vi "NISE.remote.init request string.vi"(8 "error in (no error)":errorcluster, 10 "slsc type":T1, 11 "resource":string) -> (0 "error out":errorcluster, 3 "Request String":string)   [LabVIEW 2016, in "SLSC Interface.lvclass"]
uses:
  SLSC Interface Class/SLSC Interface.lvclass
  SLSC Interface Class/NISE.slsc type.ctl
  <vilib>/NI/JSON Support for LabVIEW/JSON Data Classes/JSON Object/JSON Object.lvclass
  C:/Program Files (x86)/National Instruments/LabVIEW 2016/vi.lib/NI/JSON Support for LabVIEW/JSON Data Classes/JSON Datatype/JSON Null.lvclass
  <vilib>/NI/JSON Support for LabVIEW/JSON Data Classes/JSON Object/New JSON Object (Empty).vi
  <vilib>/NI/JSON Support for LabVIEW/JSON Data Classes/JSON Object/Insert Key Value Pair (Single String).vi
  <vilib>/NI/NI JSONRPC Server Framework/Classes/Server/Format Client Request (Auto-Increment).vi
  <vilib>/NI/NI JSONRPC Server Framework/Classes/Server/JSONRPC Server.lvclass
  <vilib>/NI/JSON Support for LabVIEW/JSON Data Classes/JSON Helper/JSON Helper.lvclass
  C:/Program Files (x86)/National Instruments/LabVIEW 2016/vi.lib/NI/JSON Support for LabVIEW/JSON Data Classes/JSON Structured Type/JSON Structure.lvclass
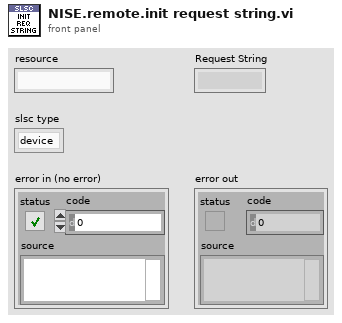
[diagram p1: front panel]
types:
  T1 = typedef "SLSC Interface.lvclass/NISE.slsc type.ctl" = enum16{"device", "nvmem", "channel", "none"}
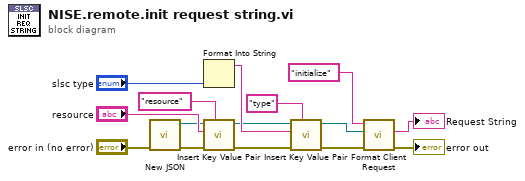
[diagram p0: block diagram]
diagram:
  n1 = call-poly <vilib>:"New JSON.vi"("error in (no error)"="error in (no error)") -> ("error out"=w9:errorcluster, "JSON Object out"=w2:refnum<class "JSON Object.lvclass">)  [unwired: 9 in]
  n2 = Format Into String("slsc type") -> (resulting string=w3:string)  [unwired: 3 in, 1 out]
  n3 = call-poly <vilib>:"Insert Key Value Pair.vi"("key"="resource" ("Name"), "error in (no error)"=w9, "value"="resource", "JSON Object in"=w2) -> ("error out"=w8:errorcluster, "JSON Object out"=w1:refnum<class "JSON Object.lvclass">)  [unwired: 5 in, 1 out]
  n4 = call-poly <vilib>:"Insert Key Value Pair.vi"("key"="type" ("Name"), "error in (no error)"=w8, "value"=w3, "JSON Object in"=w1) -> ("error out"=w12:errorcluster, "JSON Object out"=w10:refnum<class "JSON Object.lvclass">)  [unwired: 5 in, 1 out]
  n5 = call-poly <vilib>:"Format Client Request.vi"("error in (no error)"=w12, "JSON in"=w10, "method"="initialize") -> ("error out"=→"error out":errorcluster, "Request String"=→"Request String":string)  [unwired: 7 in]
